vi "Lookup Node (Name).vi"(8 "error in (no error)":errorcluster, 10 "Node Name":string, 11 "Cluster in":refnum<class "Cluster.lvclass">) -> (0 "error out":errorcluster, 2 "Node":refnum<class "Node.lvclass">, 3 "Cluster out":refnum<class "Cluster.lvclass">)   [LabVIEW 2020, in "VolatusConfig.lvlib" / "Cluster.lvclass"]
uses:
  Cluster.lvclass
  C:/dev/lv20CE/relink/lv-volatus/VolatusConfig/VolatusConfigElement/VolatusConfigElement.lvclass
  Node/Node.lvclass
  Meta Type.ctl
  VolatusConfigElement/VolatusConfigElement.lvclass/VolatusConfigElement.ctl
  VolatusConfigElement/Element.vi
  lv-cdm/CDM-Config/Config Lookup/Match Meta.vi
  lv-cdm/CDM-Config/Config Element/Owner.vi
  lv-cdm/CDM-Config/Config Manager/Lookup Descendant.vi
  lv-cdm/CDM-Config/Config Filter/Config Lookup.lvclass
  Cluster.lvclass/Cluster.ctl
  VolatusConfigElement/VolatusConfigElement.lvclass
  VolatusConfig.lvlib
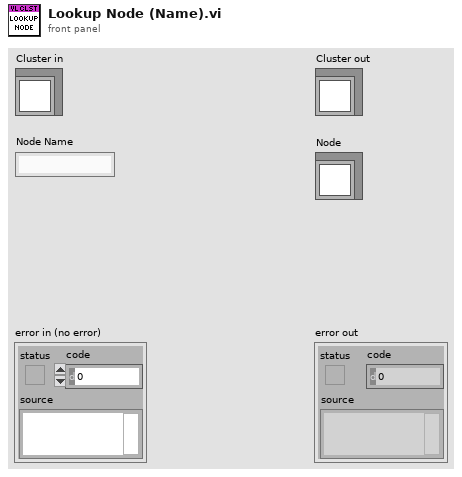
[diagram p1: front panel]
types:
  T1 = typedef "VolatusConfig.lvlib/Meta Type.ctl" = enum16{"UNKNOWN", "VL_System", "VL_Cluster", "VL_Node", "VL_Task", "VL_Group", "VL_Channel", "VL_Task_List", "VL_Scaling", "VL_Sensor", "VL_Sensor_List", "VL_Scale"}
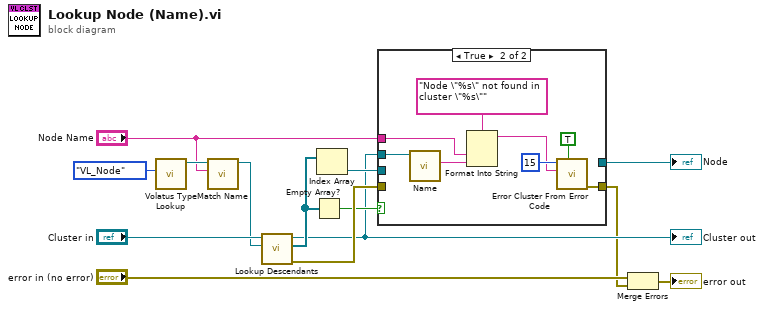
[diagram p0: block diagram]
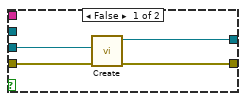
[diagram p2: hidden frame]
diagram:
  n1 = call "Volatus Type Lookup.vi"("Meta Type"=Meta_Type."VL_Node") -> ("Config Lookup out"=w11:refnum<class "Config Lookup.lvclass">)  [unwired: 9 in, 1 out]
  n2 = call "Match Name.vi"("Name"="Node Name", "Config Lookup (New)"=w11) -> ("Config Lookup out"=w10:refnum<class "Config Lookup.lvclass">)  [unwired: 8 in, 1 out]
  n3 = call "Lookup Descendants.vi"("Lookup"=w10, "VolatusConfigElement in"="Cluster in") -> ("error out"=w14:errorcluster, "Descendants"=w7:refnum<class "Config Element.lvclass">[], "VolatusConfigElement out"=w4:refnum<class "Cluster.lvclass">)  [unwired: 7 in]
  "Cluster out" <- w4
  n4 = Empty Array?(array=w7) -> (empty?=w6:bool)
  n5 = Index Array(array=w7) -> (element=w9:refnum<class "Config Element.lvclass">)  [unwired: 1 in]
  n6 = case shown="True" w6 {
    tunnel: [w18 w26] -> w2
    tunnel: w14 -> [w17 _]
    tunnel: w9 -> [w16 _]
    tunnel: [w15 _] -> w8
    tunnel: "Node Name" -> [_ w22]
    tunnel: w4 -> [_ w20]
    frame False {
      n7 = call "Create.vi"("error in (no error)"=w17, "Element"=w16) -> ("error out"=w18:errorcluster, "Node out"=w15:refnum<class "Node.lvclass">)  [unwired: 8 in]
    }
    frame True {
      n8 = call "Name.vi"("VolatusConfigElement in"=w20) -> ("Name"=w19:string)  [unwired: 8 in, 2 out]
      n9 = Format Into String(format string="Node \"%s\" not found in cluster \"%s\"", w22, w19) -> (resulting string=w21:string)  [unwired: 2 in, 1 out]
      n10 = call <vilib>:"Error Cluster From Error Code.vi"("show call chain? (False)"=TRUE, "error message (\"\")"=w21, "error code (0)"=15) -> ("error out"=w26:errorcluster)  [unwired: 6 in]
    }
  }
  "Node" <- w8
  n11 = Merge Errors("error in (no error)", w2) -> (→"error out":errorcluster)
